vi "stimulus_advanced.vi"(1 "Input Array":dbl[](array[numeric])) -> (0 "Tap Stimulus Timing Array":dbl[](array[numeric]))   [LabVIEW 2010]
panel:
  in  "stop":bool
  in  "OK Button":bool
  in  "Number of Stimulus Events":i32
  in  "Standard Deviation":dbl
  in  "Stimulus Interval":dbl
  in  "Stimulus Onset Delay":dbl
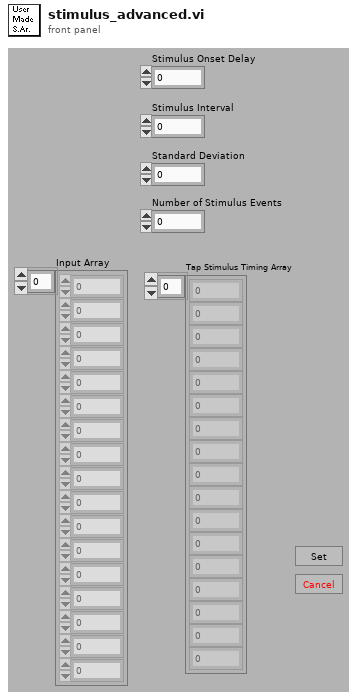
[diagram p1: front panel]
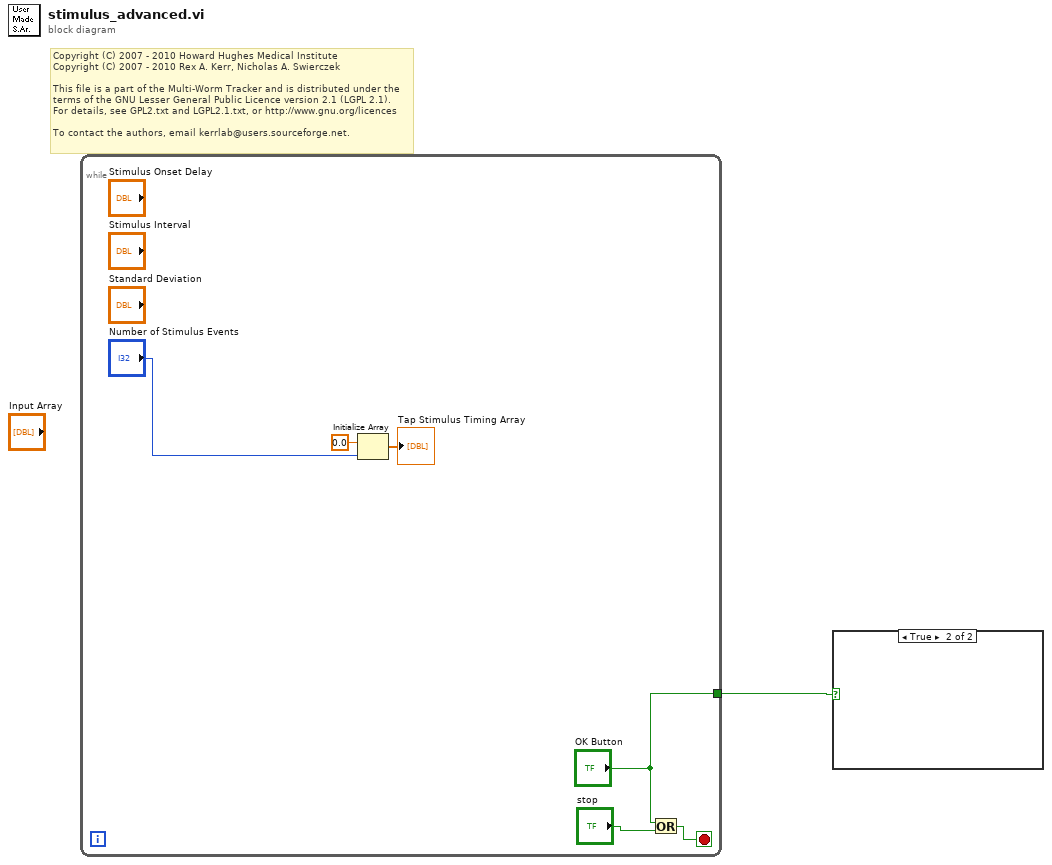
[diagram p0: block diagram]
diagram:
  # "Copyright (C) 2007 - 2010 Howard Hughes Medical Institute\nCopyright (C) 2007 - 2010 Rex A. Kerr, Nicholas A. Swierczek\n \nThis file is a part of the Multi-Worm Tracker and is distributed under the\nterms of the GNU Lesser General Public Licence version 2.1 (LGPL 2.1).\nFor details, see GPL2.txt and LGPL2.1.txt, or http://www.gnu.org/licences\n \nTo contact the authors, email kerrlab@users.sourceforge.net."
  n1 = while {
    tunnel: ["OK Button"] -> w1
    stop <- w4 stop-if-true
    n2 = Initialize Array(0.0 ("element"), "Number of Stimulus Events") -> (→"Tap Stimulus Timing Array":dbl[])
    n3 = Or(x="OK Button", y="stop") -> (x .or. y?=w4:bool)
  }
  n4 = case shown="True" w1 {
    frame False {
    }
    frame True {
    }
  }
